vi "Untitled 3.vi"   [LabVIEW 2019]
uses:
  Classes/Controller/Motion/Motion.lvclass
  Classes/Controller/Controller.lvclass
types:
  T1 = typedef "Controller.lvclass/Controllers.ctl" = cluster{"I-O.lvclass":refnum<class "I-O.lvclass">, "Motion.lvclass":refnum<class "Motion.lvclass">, "Dispenser.lvclass":refnum<class "Dispenser.lvclass">}
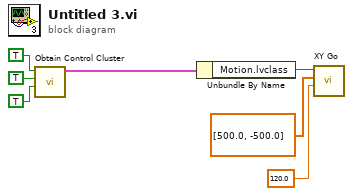
[diagram p0: block diagram]
diagram:
  n1 = call "Obtain Control Cluster.vi"("I/O"=TRUE, "Dispense"=TRUE, "Motion"=TRUE) -> ("Control Out"=w4:T1)  [unwired: 8 in]
  n2 = Unbundle By Name(w4) -> ("Motion.lvclass"=w3:refnum<class "Motion.lvclass">)
  n3 = call-dynamic "XY Go.vi"("Speed"=120.0, "XY"=dbl[] [500.0, -500.0], "Motion in"=w3) -> ()  [unwired: 7 in, 2 out]
